vi "Import Frames.vi"(8 "error in (no error)":errorcluster, 11 "Node Ptr":u64 format="%.0x") -> (0 "error out":errorcluster)   [LabVIEW 2019, in "Diagnostics Addon System Explorer.lvlib"]
uses:
  Diagnostics Addon System Explorer.lvlib
  Types/Frame.Export.ctl
  Addon Shared/Types/Signal.ctl
  Addon Shared/SubVIs/Constants.vi
  <vilib>/NI VeriStand/Custom Device API/NI VeriStand - Get Item Parent.vi
  <vilib>/NI VeriStand/Custom Device API/NI VeriStand - Get Item Data.vi
  Addon Shared/Diagnostics Addon Shared.lvlib
  <vilib>/NI VeriStand/Custom Device Tools/Custom Device Utility Library/Custom Device Utility Library.lvlib
  <vilib>/NI VeriStand/Custom Device API/Custom Device API.lvlib
panel:
  in  "Tag":string
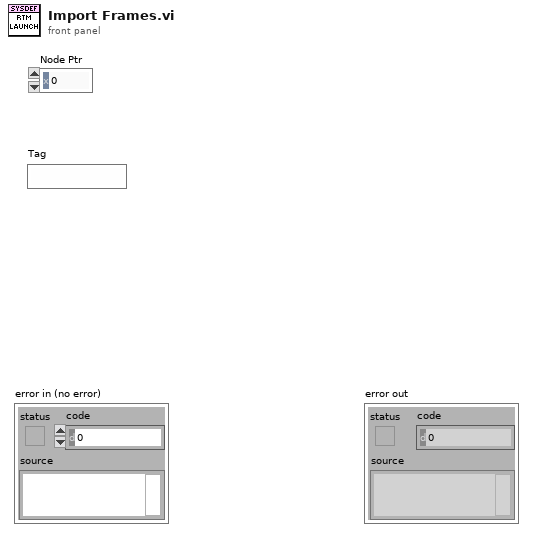
[diagram p1: front panel]
types:
  T1 = typedef "Diagnostics Addon System Explorer.lvlib/Frame.Export.ctl" = cluster{"Name":string, "ID":u32, "Signals":T2[]}
  T2 = typedef "Diagnostics Addon Shared.lvlib/Signal.ctl" = cluster{"Start Bit":u32, "Length":u32, "Scaling Factor":dbl, "Scaling Offset":dbl, "Minimum":dbl, "Maximum":dbl, "Data Type":u32, "Byte Order":u32, "Default Value":dbl, "Name":string, "Units":string}
  T3 = typedef "Custom Device API.lvlib/Custom Device Item Ref.ctl" = u64
  T4 = typedef "Diagnostics Addon Shared.lvlib/Type.ctl" = enum16{"DID", "CDID", "PID", "CPID", "Read Memory", "Write Memory", "IO Control", "Routine Start", "Routine Request", "Routine Stop", "User Defined", "DTC Control", "Clear DTCs", "Read DTCs", "Start DTCs", "DTC Change Count", "Tester Present", "Unlock ECU", "Reset ECU", "Diag Session Control", "Communication Control", "DPID Control", "Poll Control", "Diag CAN Control"}
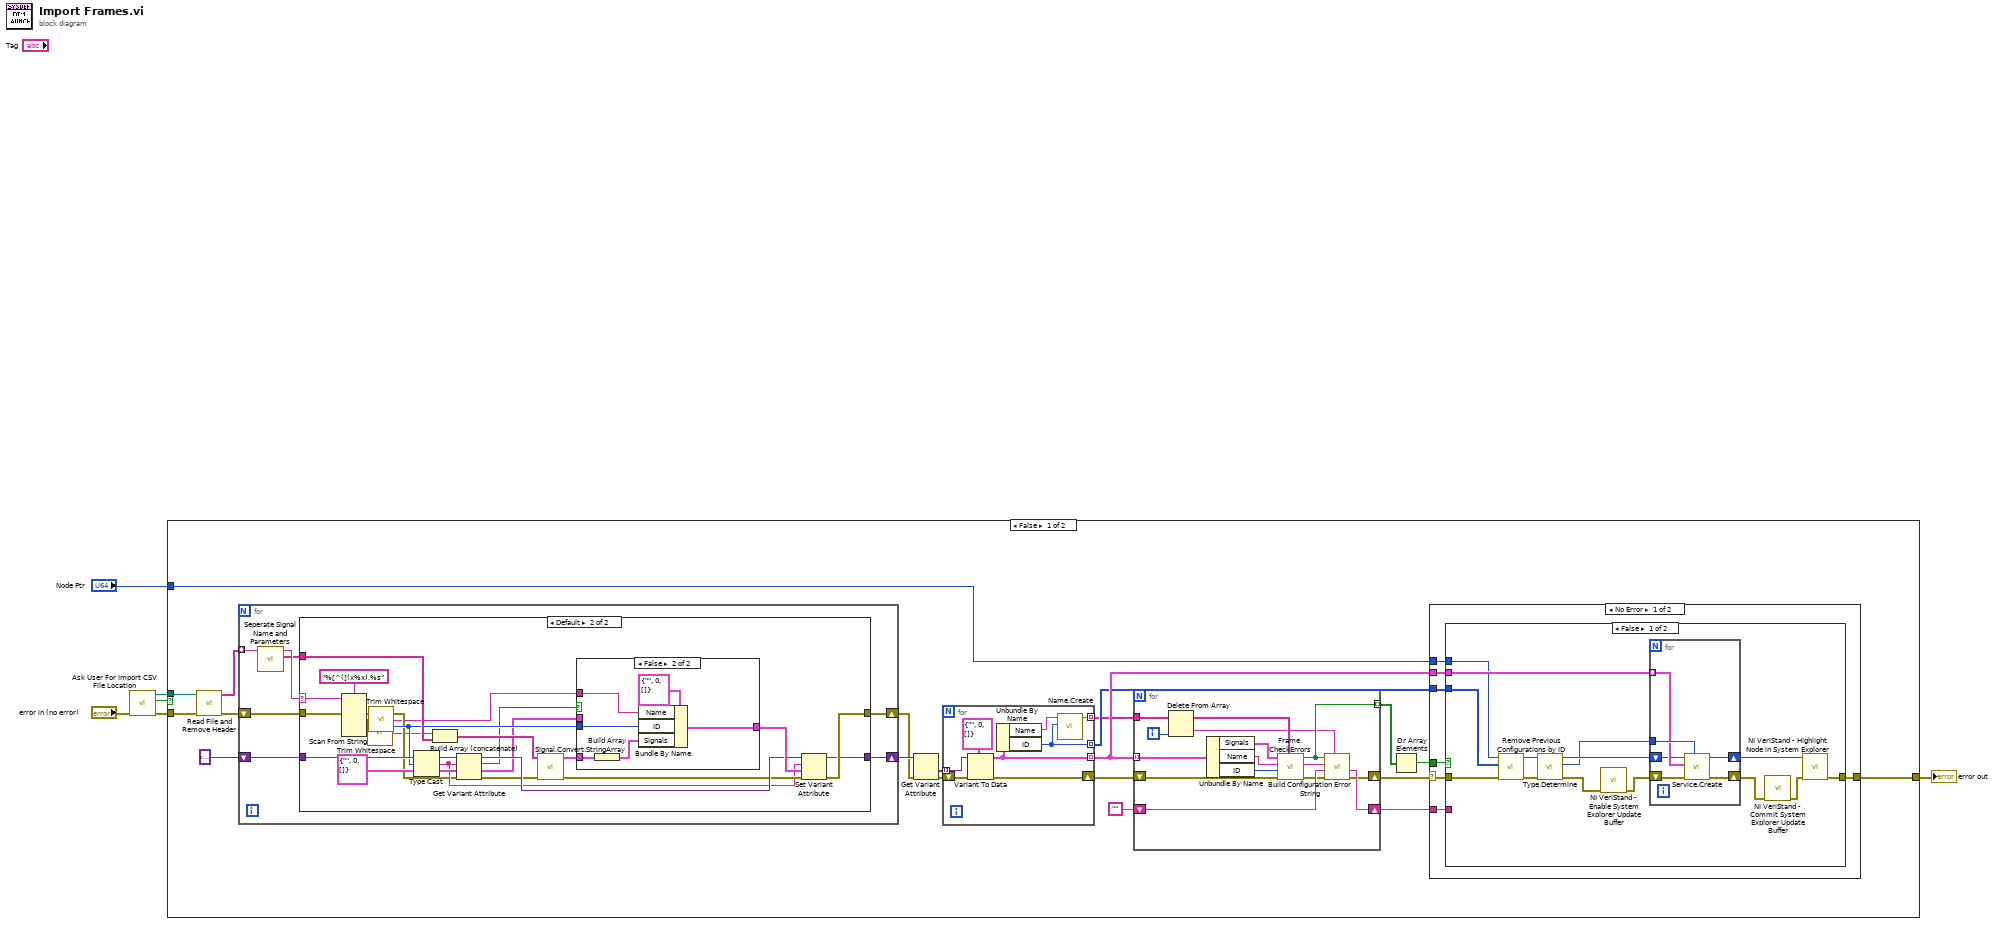
[diagram p0: block diagram]
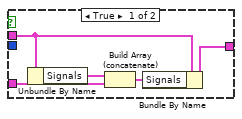
[diagram p3: hidden frame]
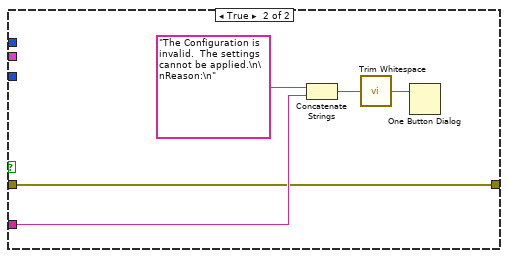
[diagram p4: hidden frame]
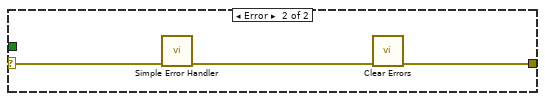
[diagram p5: hidden frame]
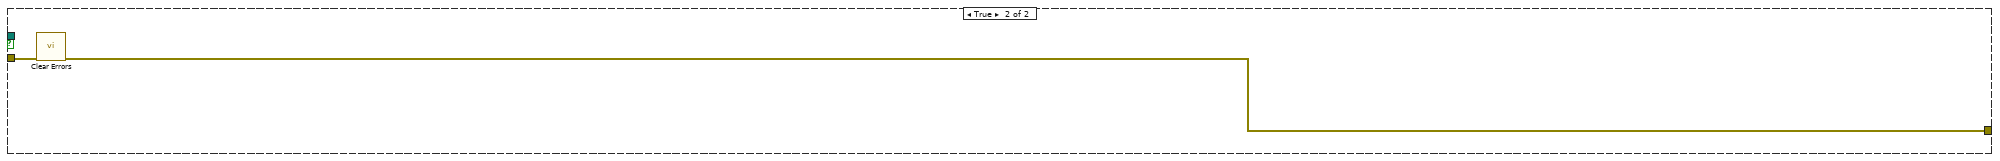
[diagram p6: hidden frame]
diagram:
  n1 = call "Ask User For Import CSV File Location.vi"("error in (no error)"="error in (no error)") -> ("error out"=w5:errorcluster, "cancelled"=w6:bool, "selected path"=w4:path)  [unwired: 8 in]
  n2 = case shown="False" w6 {
    tunnel: w5 -> [w26 w129]
    tunnel: w4 -> [w25 _]
    tunnel: "Node Ptr" -> [w11 _]
    tunnel: [w13 w128] -> w2
    frame False {
      n3 = call "Read File and Remove Header.vi"("error in (no error)"=w26, "selected path"=w25) -> ("error out"=w24:errorcluster, "Array"=w8:string[])  [unwired: 8 in]
      n4 = for {
        tunnel: w8 -> [w33] mode=indexing
        shift-right: [w30] -> w21
        shift-left: w24 -> [w31]
        shift-right: [w29] -> w22
        shift-left: variant -> [w32]
        n5 = call "Seperate Signal Name and Parameters.vi"("String"=w33) -> ("Signal Parameters"=w27:string[], "Signal Name"=w28:string)  [unwired: 9 in]
        n6 = case shown="Default" w28 {
          selector: w28 -> [_ w39]
          tunnel: w27 -> [_ w58]
          tunnel: w32 -> [w35 w53]
          tunnel: w31 -> [w34 w52]
          tunnel: [w34 w46] -> w30
          tunnel: [w35 w45] -> w29
          frame "" {
          }
          frame Default {
            n7 = Scan From String(format string="%[^(](x%x).%s", input string=w39, error in=w52) -> (error out=w43:errorcluster, output 1=w56:string, output 2=w50:u32, output 3=w54:string)  [unwired: 4 in, 2 out]
            n8 = call <vilib>:"Trim Whitespace.vi"("string"=w54) -> ("trimmed string"=w36:string)  [unwired: 1 in]
            n9 = call <vilib>:"Trim Whitespace.vi"("string"=w56) -> ("trimmed string"=w37:string)  [unwired: 1 in]
            n10 = Type Cast(x=w50) -> (*(type *) &x=w44:string)  [unwired: 1 in]
            n11 = Build Array (concatenate)(w36, w58) -> (w55:string[])
            n12 = Get Variant Attribute(Variant=w53, name=w44, default value (empty Variant)=T1 {"Name"="", "ID"=0, "Signals"=[]} ("DIDPID"), error in=w43) -> (duplicate Variant=w48:variant, found=w41:bool, value=w40:T1, error out=w42:errorcluster)
            n13 = call "Signal.Convert.StringArray.vi"("error in (no error)"=w42, "Signal Parameters"=w55) -> ("error out"=w47:errorcluster, "Signal Parameters"=w57:T2)  [unwired: 8 in]
            n14 = case shown="False" w41 {
              tunnel: w57 -> [w61 w68]
              tunnel: w37 -> [_ w67]
              tunnel: w50 -> [_ w65]
              tunnel: [w59 w64] -> w49
              tunnel: w40 -> [w63 _]
              frame True {
                n15 = Unbundle By Name(w63) -> ("Signals"=w62:T2[])
                n16 = Build Array (concatenate)(w62, w61) -> (w60:T2[])
                n17 = Bundle By Name(cluster=w63, "Signals"=w60) -> (w59:T1)
              }
              frame False {
                n18 = Build Array(w68) -> (w66:T2[])
                n19 = Bundle By Name(cluster=T1 {"Name"="", "ID"=0, "Signals"=[]} ("DIDPID"), "Name"=w67, "ID"=w65, "Signals"=w66) -> (w64:T1)
              }
            }
            n20 = Set Variant Attribute(Variant=w48, name=w44, value=w49, error in=w47) -> (Variant out=w45:variant, error out=w46:errorcluster)  [unwired: 1 out]
          }
        }
      }
      n21 = Get Variant Attribute(Variant=w22, error in=w21) -> (values=w20:variant[], error out=w19:errorcluster)  [unwired: 2 in, 2 out]
      n22 = for {
        tunnel: w20 -> [w76] mode=indexing
        shift-right: [w74] -> w12
        shift-left: w19 -> [w75]
        tunnel: [w73] -> w14 mode=indexing
        tunnel: [w72] -> w10 mode=indexing
        tunnel: [w70] -> w7 mode=indexing
        n23 = Variant To Data(error in=w75, type=T1 {"Name"="", "ID"=0, "Signals"=[]} ("DIDPID"), Variant=w76) -> (data=w73:T1, error out=w74:errorcluster)
        n24 = Unbundle By Name(w73) -> ("Name"=w71:string, "ID"=w72:u32)
        n25 = call "Name.Create.vi"("PID Number"=w72, "PID Name"=w71) -> ("VS Name"=w70:string)  [unwired: 9 in]
      }
      n26 = for {
        tunnel: w14 -> [w92] mode=indexing
        shift-right: [w78] -> w9
        shift-left: w12 -> [w88]
        shift-right: [w79] -> w15
        shift-left: "" -> [w82]
        tunnel: [w84] -> w17 mode=indexing
        tunnel: w7 -> [w87]
        i -> [w86]
        n27 = Delete From Array(array=w87, index=w86) -> (deleted portion=w81:string, array with subset deleted=w85:string[])  [unwired: 1 in]
        n28 = Unbundle By Name(w92) -> ("Signals"=w89:T2[], "Name"=w91:string, "ID"=w90:u32)
        n29 = call "Frame.CheckErrors.vi"("Existing PIDs"=w85, "error in (no error)"=w88, "ID"=w90, "Name"=w91, "Signals"=w89) -> ("error out"=w80:errorcluster, "Error Type"=w83:string, "Error?"=w84:bool)  [unwired: 4 in]
        n30 = call "Build Configuration Error String.vi"("Name"=w81, "error in (no error)"=w80, "String in"=w82, "Error"=w83, "Error?"=w84) -> ("error out"=w78:errorcluster, "String out"=w79:string)  [unwired: 5 in]
      }
      n31 = Or Array Elements(Boolean array=w17) -> (logical OR=w16:bool)
      n32 = case shown="No Error" w9 {
        selector: w9 -> [w95 w127]
        tunnel: w16 -> [w99 _]
        tunnel: w15 -> [w98 _]
        tunnel: w14 -> [w97 _]
        tunnel: [w96 w125] -> w13
        tunnel: w11 -> [w94 _]
        tunnel: w10 -> [w93 _]
        frame No Error {
          n33 = case shown="False" w99 {
            tunnel: w98 -> [_ w122]
            tunnel: w95 -> [w103 w121]
            tunnel: w97 -> [w109 _]
            tunnel: [w108 w121] -> w96
            tunnel: w94 -> [w104 _]
            tunnel: w93 -> [w102 _]
            frame False {
              n34 = call "Remove Previous Configurations by ID.vi"("error in (no error)"=w103, "Imported IDs"=w102, "Node In"=w104) -> ("error out"=w101:errorcluster, "Node Out"=w100:T3)  [unwired: 7 in]
              n35 = call "Type.Determine.vi"("error in (no error)"=w101, "Node Ptr"=w100) -> ("error out"=w107:errorcluster, "Type"=w105:T4, "Item Ref out"=w106:T3)  [unwired: 6 in, 1 out]
              n36 = call <vilib>:"NI VeriStand - Enable System Explorer Update Buffer.vi"("error in (no error)"=w107) -> ("error out"=w112:errorcluster)  [unwired: 10 in]
              n37 = for {
                shift-right: [w115] -> w111
                shift-left: w112 -> [w114]
                shift-right: [w116] -> w113
                shift-left: w106 -> [w117]
                tunnel: w109 -> [w118] mode=indexing
                tunnel: w105 -> [w119]
                n38 = call "Service.Create.vi"("Type"=w119, "error in (no error)"=w114, "Variant"=w118, "Section Ptr"=w117) -> ("error out"=w115:errorcluster, "Parent Ref out"=w116:T3)  [unwired: 6 in]
              }
              n39 = call <vilib>:"NI VeriStand - Commit System Explorer Update Buffer.vi"("error in (no error)"=w111) -> ("error out"=w110:errorcluster)  [unwired: 10 in]
              n40 = call <vilib>:"NI VeriStand - Highlight Node in System Explorer.vi"("error in (no error)"=w110, "Item Ref in"=w113) -> ("error out"=w108:errorcluster)  [unwired: 8 in, 1 out]
            }
            frame True {
              n41 = Concatenate Strings("The Configuration is invalid.  The settings cannot be applied.\n\nReason:\n" ("message"), w122) -> (w124:string)
              n42 = call <vilib>:"Trim Whitespace.vi"("string"=w124) -> ("trimmed string"=w120:string)  [unwired: 1 in]
              n43 = One Button Dialog(message=w120) -> ()  [unwired: 1 in, 1 out]
            }
          }
        }
        frame Error {
          n44 = call <vilib>:"Simple Error Handler.vi"("error in (no error)"=w127) -> ("error out"=w126:errorcluster)  [unwired: 4 in, 4 out]
          n45 = call <vilib>:"Clear Errors.vi"("error in (no error)"=w126) -> ("error out"=w125:errorcluster)  [unwired: 5 in, 1 out]
        }
      }
    }
    frame True {
      n46 = call <vilib>:"Clear Errors.vi"("error in (no error)"=w129) -> ("error out"=w128:errorcluster)  [unwired: 5 in, 1 out]
    }
  }
  "error out" <- w2
